vi "finalusedAOhack.vi"(1 "presorted indices":u32[](array[numeric])) -> (0 "AO wf out":waveform(dbl)[](array[waveform]))   [LabVIEW 2015]
uses:
  Objects/configuration.vi
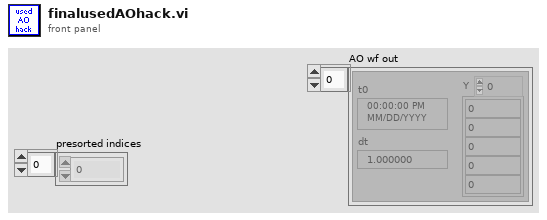
[diagram p1: front panel]
types:
  T1 = typedef "LVRectTypeDef.ctl" = cluster{"Left":i16, "Top":i16, "Right":i16, "Bottom":i16}
  T2 = cluster{"Xpixels":i32, "Vxminref":dbl, "Vxmaxref":dbl, "P":dbl, "Ypixels":i32, "Vyminref":dbl, "Vymaxref":dbl, "srate":sgl, "sAOxy":i32, "timeout":dbl, "type":string, "date":string, "time":string, "Colormap":u16, "Drawing Mode":u16, "Scanning Mode":u16, "square pixels":bool, "square matrix":bool, "Xpixels Img":i32, "Vx-min Img":dbl, "VX-max Img":dbl, "Ypixels Img":i32, "Vy-min Img":dbl, "Vy-max Img ":dbl, "Angle Img":dbl, "autoshutter":bool, "finite":bool, "cont":bool, "wavdet":bool, "measpoints":i32, "avpp":i32, "bufferAO":i32, "bufferAI":i32, "starttick":u32, "waveform":path, "Vx-ref":dbl, "Vy-ref":dbl, "refreshrate":dbl, "refreshbuffer":i32, "tt_cycles":i32, "motorref":refnum<k7>, "mirrorswitch":refnum<k7>, "sample mode":i32, "maxbufferAI":i32, "srateAODO":sgl, "bin":sgl, "Pel":sgl, "Angle draw":dbl, "srate Img":sgl, "ROIimg_plotbounds":T1, "auto OD":bool, "ODfilt":u16, "aAI":i32[], "aCI":i32[], "aAO":u32[], "aDO":u32[], "refwfsize":dbl, "Lifetime":bool, "Vz-Img":dbl, "Vz-ref":dbl, "Vz-reset":dbl, "AIoverride":bool, "aAS":u32[], "XYZstart":dbl[]}
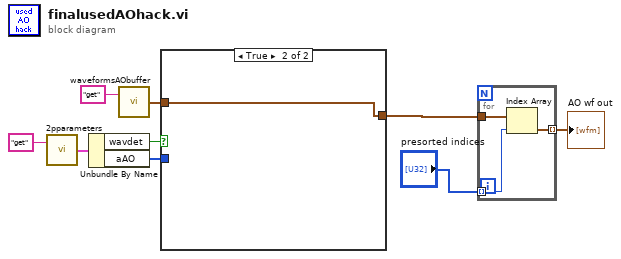
[diagram p0: block diagram]
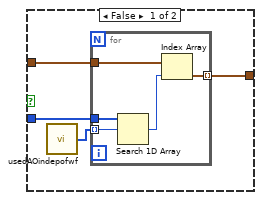
[diagram p2: hidden frame]
diagram:
  n1 = call "2pparameters.vi"("command"="get") -> ("params out"=w7:T2)  [unwired: 1 in]
  n2 = Unbundle By Name(w7) -> ("wavdet"=w5:bool, "aAO"=w6:u32[])
  n3 = call "waveformsAObuffer.vi"("command"="get") -> ("AO wf out"=w4:waveform(dbl)[])  [unwired: 1 in]
  n4 = case shown="True" w5 {
    tunnel: w6 -> [w13 _]
    tunnel: w4 -> [w12 w19]
    tunnel: [w11 w19] -> w2
    frame False {
      n5 = call "usedAOindepofwf.vi"() -> ("AO"=w10:i32[])  [unwired: 1 in]
      n6 = for {
        tunnel: w10 -> [w18] mode=indexing
        tunnel: w13 -> [w17]
        tunnel: w12 -> [w15]
        tunnel: [w14] -> w11 mode=indexing
        n7 = Search 1D Array(1D array=w17, element=w18) -> (index of element=w16:i32)  [unwired: 1 in]
        n8 = Index Array(array=w15, index=w16) -> (element=w14:waveform(dbl))
      }
    }
    frame True {
    }
  }
  n9 = for {
    tunnel: "presorted indices" -> [w21] mode=indexing
    tunnel: w2 -> [w22]
    tunnel: [w20] -> w1 mode=indexing
    n10 = Index Array(array=w22, index=w21) -> (element=w20:waveform(dbl))
  }
  "AO wf out" <- w1
